vi "getStep.vi"(1 "Radio Buttons":enum32{"Coarse (mm) ", "Fine (um) "}(radio)=enum."Fine (um) ") -> (0 "step":dbl)   [LabVIEW 2015]
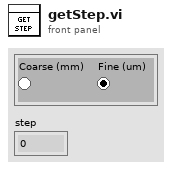
[diagram p1: front panel]
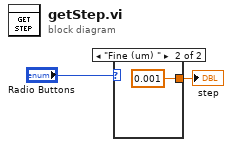
[diagram p0: block diagram]
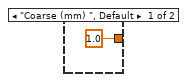
[diagram p2: hidden frame]
diagram:
  n1 = case shown="\"Fine (um) \"" "Radio Buttons" {
    tunnel: [1.0 0.001] -> w1
    frame "Coarse (mm) ", Default {
    }
    frame "Fine (um) " {
    }
  }
  "step" <- w1
